vi "RSZVB Get External Signal Generator Output.vi"(8 "error in (no error)":errorcluster {"code" format="%.0x"}, 10 "Channel (1)":i32=1, 11 "VISA session":refnum<visa-resource-name>) -> (0 "error out":errorcluster {"code" format="%.0x"}, 1 "Ext Signal Generator Output":bool, 3 "dup VISA session":refnum<visa-resource-name>)   [LabVIEW 2011]
doc: "This VI returns either the R&S ZVA pulse generator signals or the external pulse generator signals to the PULSE GENERATOR OUT connector.\n\nRemote-control command(s):\n[SENSe<Ch>:]EUNit:PGENerator:OUTPut:EXTernal?"
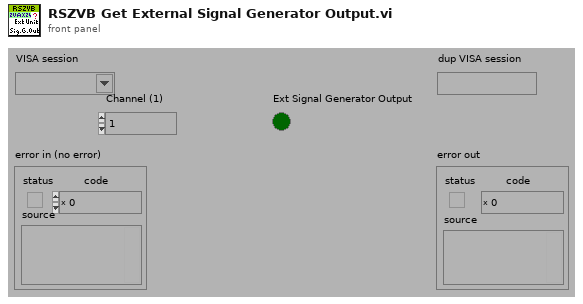
[diagram p1: front panel]
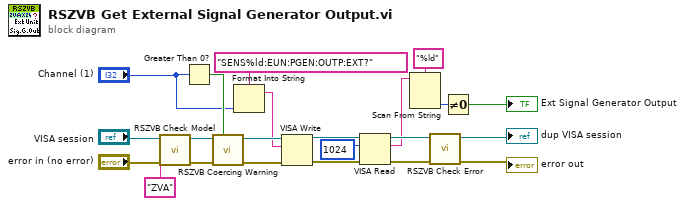
[diagram p0: block diagram]
diagram:
  n1 = call "RSZVB Check Model.vi"("error in (no error)"="error in (no error)", "Model"="ZVA" ("Options"), "VISA session"="VISA session") -> ("error out"=w7:errorcluster, "dup VISA session"=w8:refnum<visa-resource-name>)  [unwired: 7 in]
  n2 = Greater Than 0?(x="Channel (1)") -> (x > 0?=w17:bool)
  n3 = call "RSZVB Coercing Warning.vi"("In Range?"=w17, "error in (no error)"=w7, "VISA session"=w8) -> ("error out"=w20:errorcluster, "dup VISA session"=w21:refnum<visa-resource-name>)  [unwired: 7 in]
  n4 = Format Into String(format string="SENS%ld:EUN:PGEN:OUTP:EXT?", "Channel (1)") -> (resulting string=w19:string)  [unwired: 2 in, 1 out]
  n5 = VISA Write(VISA resource name=w21, write buffer=w19, error in (no error)=w20) -> (VISA resource name out=w9:refnum<visa-resource-name>, error out=w11:errorcluster)  [unwired: 1 out]
  n6 = VISA Read(VISA resource name=w9, byte count=u32 1024 ("byte count (0)"), error in (no error)=w11) -> (VISA resource name out=w16:refnum<visa-resource-name>, read buffer=w14:string, error out=w15:errorcluster)  [unwired: 1 out]
  n7 = Scan From String(format string="%ld", input string=w14) -> (output 1=w12:i32)  [unwired: 3 in, 3 out]
  n8 = call "RSZVB Check Error.vi"("error in (no error)"=w15, "VISA session"=w16) -> ("error out"=→"error out":errorcluster, "dup VISA session"=→"dup VISA session":refnum<visa-resource-name>)  [unwired: 8 in]
  n9 = Not Equal To 0?(x=w12) -> (x != 0?=→"Ext Signal Generator Output":bool)
